vi "TintAndShade.vi"(1 "Operation":string(combo), 2 "Concentration":dbl(slide)=0.001 min=0.001 max=0.999 step=0.0001 scale=0.0001..0.999, 3 "Reflectance":dbl[](array[numeric])) -> (0 "Resultant Color":dbl[](array[numeric]))   [LabVIEW 2013]
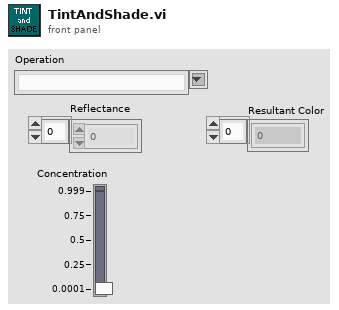
[diagram p1: front panel]
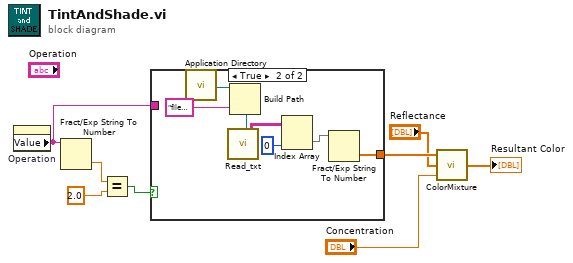
[diagram p0: block diagram]
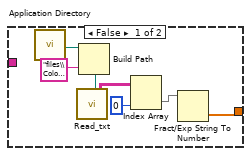
[diagram p2: hidden frame]
diagram:
  n1 = property on="Operation" class="CmbBox"() -> ("Value"=w6:string)  [unwired: 2 in, 2 out]
  n2 = Fract/Exp String To Number(string=w6) -> (number=w8:dbl)  [unwired: 3 in, 1 out]
  n3 = Equal?(x=w8, y=2.0) -> (x = y?=w1:bool)
  n4 = case shown="True" w1 {
    tunnel: [w9 w16] -> w5
    tunnel: w6 -> [_ _]
    frame False {
      n5 = call <vilib>:"Application Directory.vi"() -> ("Application Directory"=w10:path)
      n6 = Build Path(base path=w10, name or relative path="files\\Colors\\White.txt") -> (appended path=w12:path)
      n7 = call "Read_txt.vi"("file path (dialog if empty)"=w12) -> ("Elements"=w13:string[][])  [unwired: 2 out]
      n8 = Index Array(array=w13, index (col)=0 ("index (row)")) -> (element=w14:string[])  [unwired: 1 in]
      n9 = Fract/Exp String To Number(string=w14) -> (number=w9:dbl[])  [unwired: 3 in, 1 out]
    }
    frame True {
      n10 = call <vilib>:"Application Directory.vi"() -> ("Application Directory"=w17:path)
      n11 = Build Path(base path=w17, name or relative path="files\\Colors\\Black.txt") -> (appended path=w19:path)
      n12 = call "Read_txt.vi"("file path (dialog if empty)"=w19) -> ("Elements"=w20:string[][])  [unwired: 2 out]
      n13 = Index Array(array=w20, index (col)=0 ("index (row)")) -> (element=w21:string[])  [unwired: 1 in]
      n14 = Fract/Exp String To Number(string=w21) -> (number=w16:dbl[])  [unwired: 3 in, 1 out]
    }
  }
  n15 = call "ColorMixture.vi"("Concentration1"="Concentration", "Reflectance spectrum 2"="Reflectance", "Reflectance spectrum"=w5) -> ("Mixtured colors"=→"Resultant Color":dbl[])
